vi "Create.vi"(8 "Error In":errorcluster, 10 "Tag":string, 11 "Animation In":refnum<class "Animation.lvclass">) -> (0 "Error Out":errorcluster, 3 "Animation Out":refnum<class "Animation.lvclass">)   [LabVIEW 2021, in "Animation.lvclass"]
uses:
  Animation.lvclass
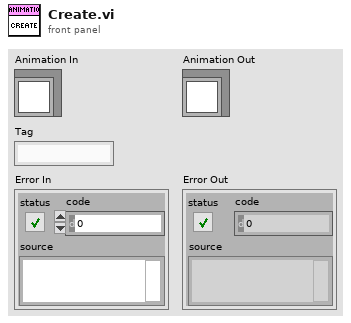
[diagram p1: front panel]
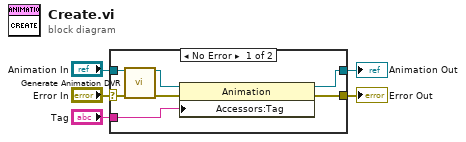
[diagram p0: block diagram]
diagram:
  n1 = case shown="No Error" "Error In" {
    selector: "Error In" -> [w12 w14]
    tunnel: [w7 w14] -> w4
    tunnel: [w8 w13] -> w3
    tunnel: "Animation In" -> [w11 w13]
    tunnel: "Tag" -> [w6 _]
    frame No Error {
      n2 = call "Generate Animation DVR.vi"("Error In"=w12, "Animation In"=w11) -> ("Error Out"=w9:errorcluster, "Animation Out"=w10:refnum<class "Animation.lvclass">)  [unwired: 8 in]
      n3 = property class="Animation"(reference=w10, error in=w9, "Accessors:Tag"=w6) -> (reference out=w8:refnum<class "Animation.lvclass">, error out=w7:errorcluster)
    }
    frame Error {
    }
  }
  "Animation Out" <- w3
  "Error Out" <- w4
